vi "Set Error (ID).vi"(8 "error in (no error)":errorcluster, 9 "attributes":string[](array[string]), 10 "new error":T1, 11 "error list <owner> in":variant) -> (0 "error out":errorcluster, 3 "error list <owner> out":variant)   [LabVIEW 2017]
uses:
  Error File Management/Controls/NI Error.ctl
  Attributes.vi
  Error File Management/Error File Management.lvlib
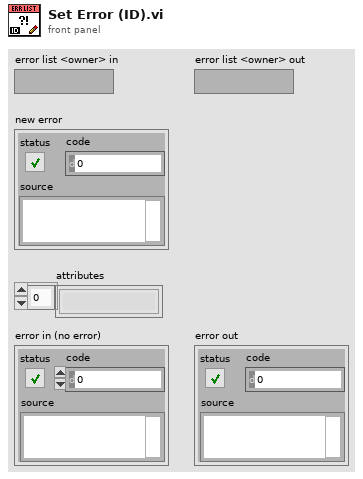
[diagram p1: front panel]
types:
  T1 = typedef "Error File Management.lvlib/NI Error.ctl" = errorcluster
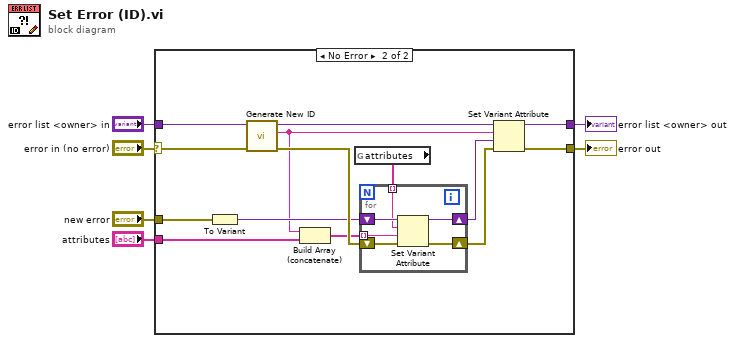
[diagram p0: block diagram]
diagram:
  n1 = case shown="No Error" "error in (no error)" {
    selector: "error in (no error)" -> [w8 w13]
    tunnel: "new error" -> [_ w21]
    tunnel: "error list <owner> in" -> [w7 w16]
    tunnel: [w7 w20] -> w4
    tunnel: [w8 w19] -> w2
    tunnel: "attributes" -> [_ w15]
    frame Error {
    }
    frame No Error {
      n2 = To Variant(anything=w21) -> (Variant=w18:variant)
      n3 = call "Generate New ID.vi"("error in (no error)"=w13, "error list in"=w16) -> ("error out"=w22:errorcluster, "new ID"=w10:string, "error list out"=w17:variant)  [unwired: 7 in]
      n4 = Build Array (concatenate)(w10, w15) -> (w11:string[])
      n5 = global read "Attributes.vi" "attributes"() -> (w9:string[])
      n6 = for {
        shift-right: [w26] -> w12
        shift-left: w22 -> [w28]
        shift-right: [w25] -> w14
        shift-left: w18 -> [w27]
        tunnel: w9 -> [w24] mode=indexing
        tunnel: w11 -> [w23] mode=indexing
        n7 = Set Variant Attribute(Variant=w27, name=w24, value=w23, error in=w28) -> (Variant out=w25:variant, error out=w26:errorcluster)  [unwired: 1 out]
      }
      n8 = Set Variant Attribute(Variant=w17, name=w10, value=w14, error in=w12) -> (Variant out=w20:variant, error out=w19:errorcluster)  [unwired: 1 out]
    }
  }
  "error list <owner> out" <- w4
  "error out" <- w2
